vi "_s_Bronkhorst Serial Module.vi"(5 "Module (T:Enable)":bool=TRUE, 6 "Mode (T:Digital)":bool=TRUE, 7 "Command":T1=enum."Request Serial Number", 8 "error in (no error)":errorcluster, 9 "Setpoint %":dbl, 10 "Nodo":u8=3, 11 "VISA resource name":refnum<visa-resource-name>="COM1") -> (0 "error out":errorcluster, 1 "Reading":T2, 2 "Result":string, 3 "Value":string)   [LabVIEW 2013]
uses:
  _s_Bronkhorst Control.ctl
  <vilib>/Instr/_visa.llb/VISA Configure Serial Port (Instr).vi
panel:
  out "ReadString":string
  out "Bytes?":u32
  out "SendString":string
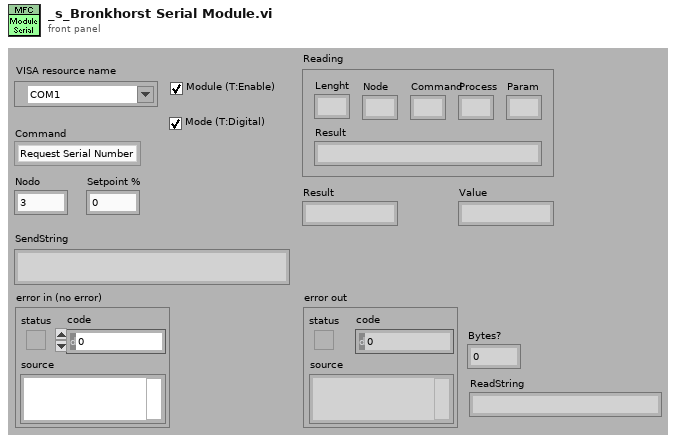
[diagram p1: front panel]
types:
  T1 = typedef "_s_Bronkhorst Control.ctl" = enum16{"Inicializar", "Request IdnString", "Request Serial Number", "Request Fluid Number", "Request Fluid Name", "Request Sensor Type", "Request Cap 0", "Request Cap100", "Request Units", "Request CapUnitStr", "Request Setpoint %", "Request Setpoint", "Request Measure %", "Request Measure ", "Send Control Mode", "Send Fluid Number", "Send Setpoint %", "Send Setpoint", "Shutdown"}
  T2 = cluster{"Lenght":string, "Node":string, "Process":string, "Param":string, "Command":string, "Result":string}
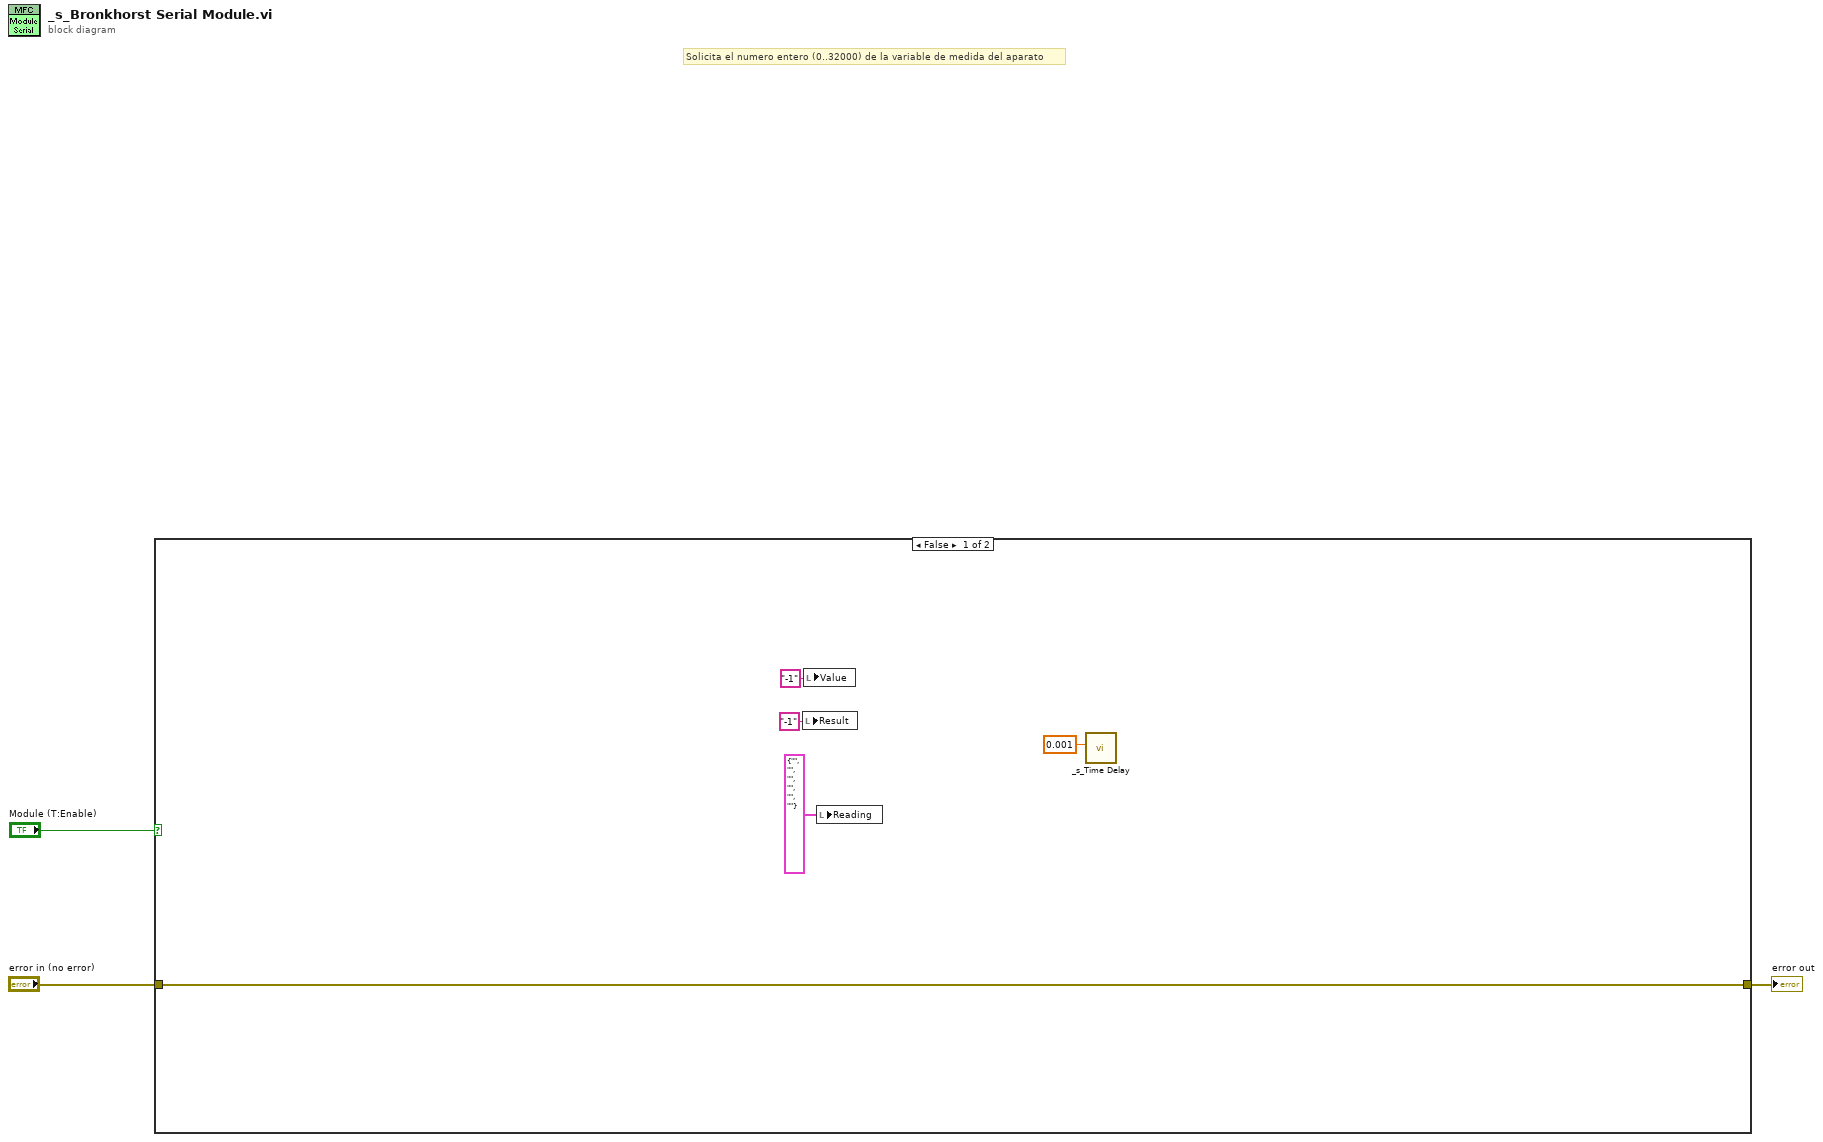
[diagram p0: block diagram]
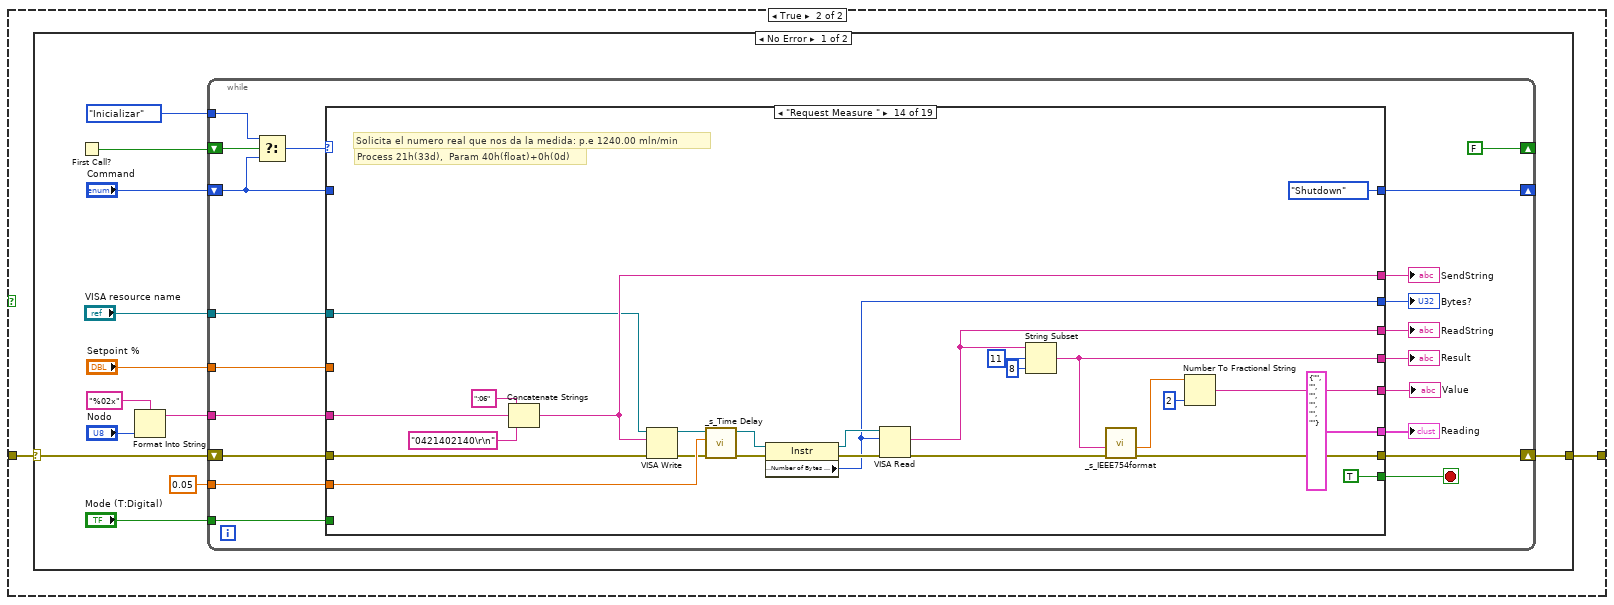
[diagram p2: hidden frame]
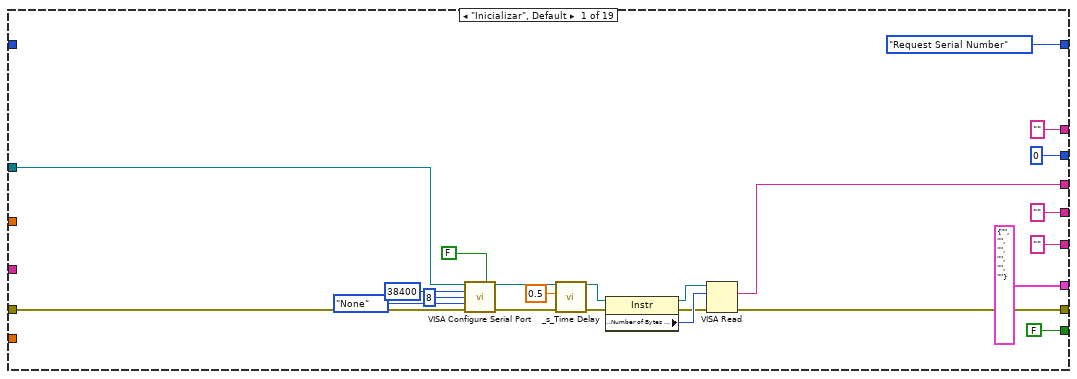
[diagram p3: hidden frame]
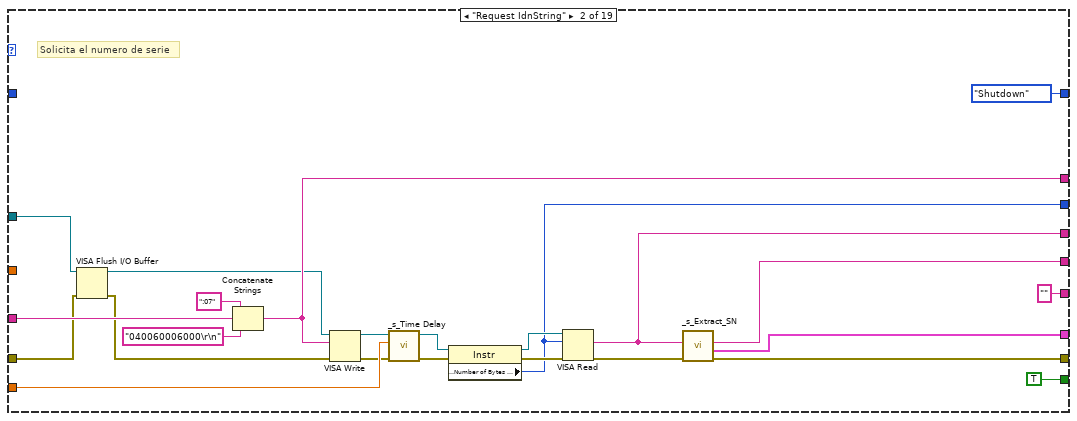
[diagram p4: hidden frame]
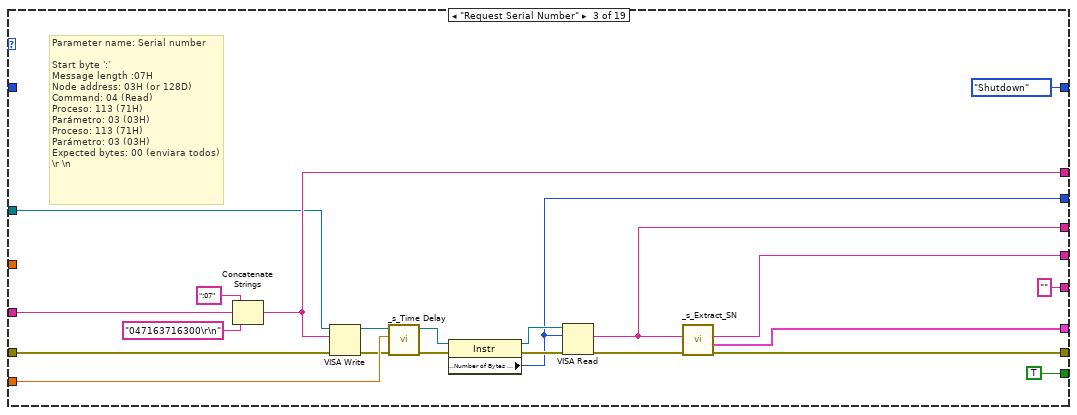
[diagram p5: hidden frame]
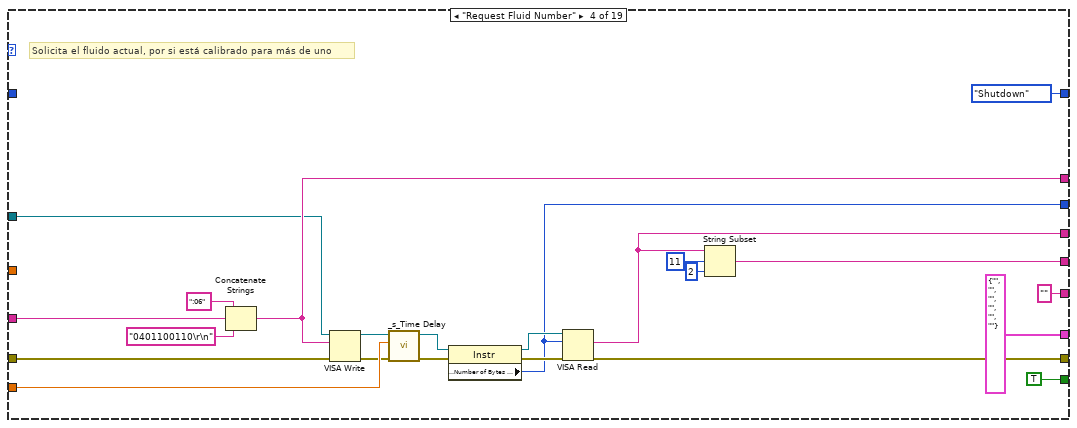
[diagram p6: hidden frame]
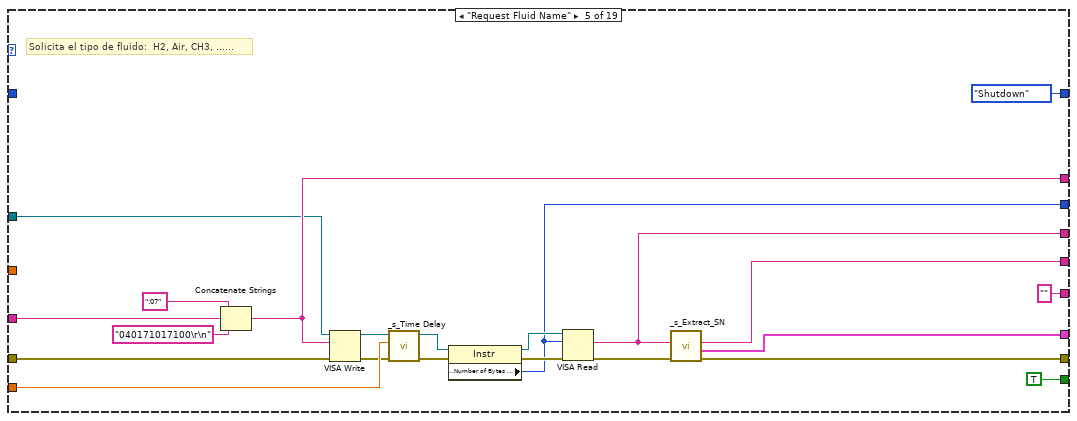
[diagram p7: hidden frame]
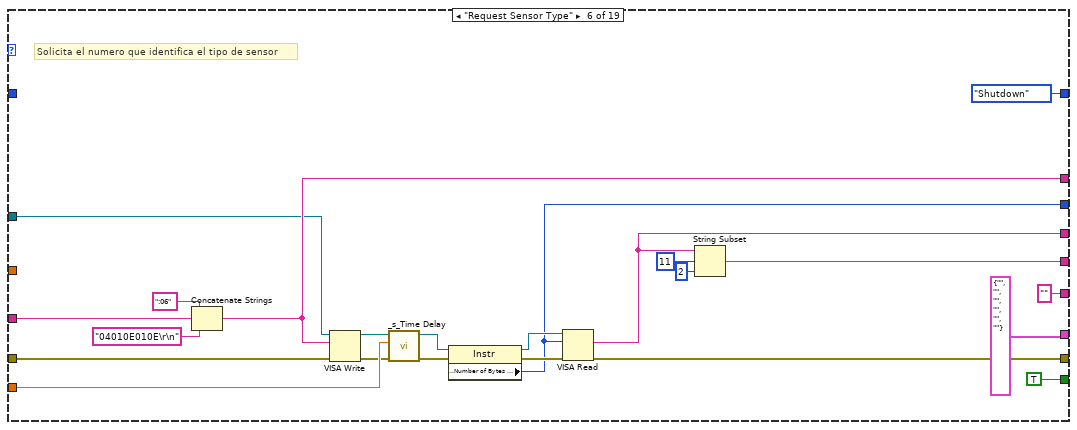
[diagram p8: hidden frame]
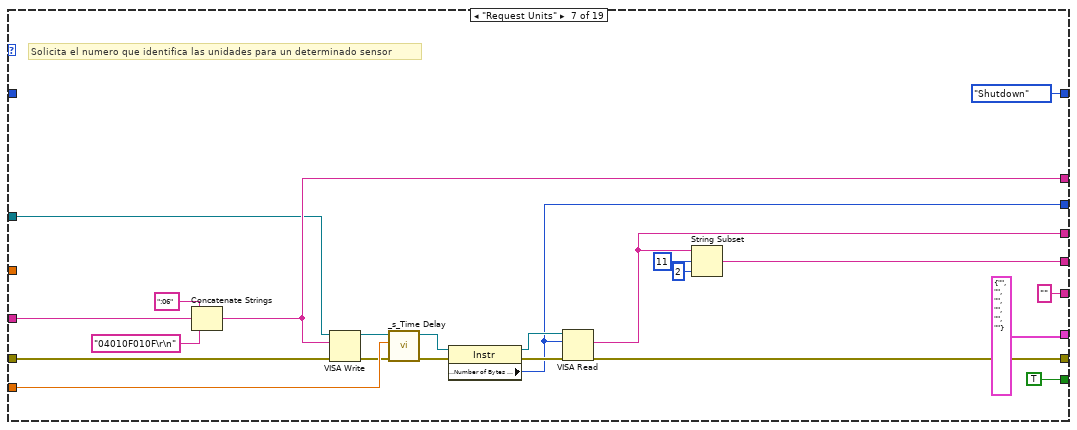
[diagram p9: hidden frame]
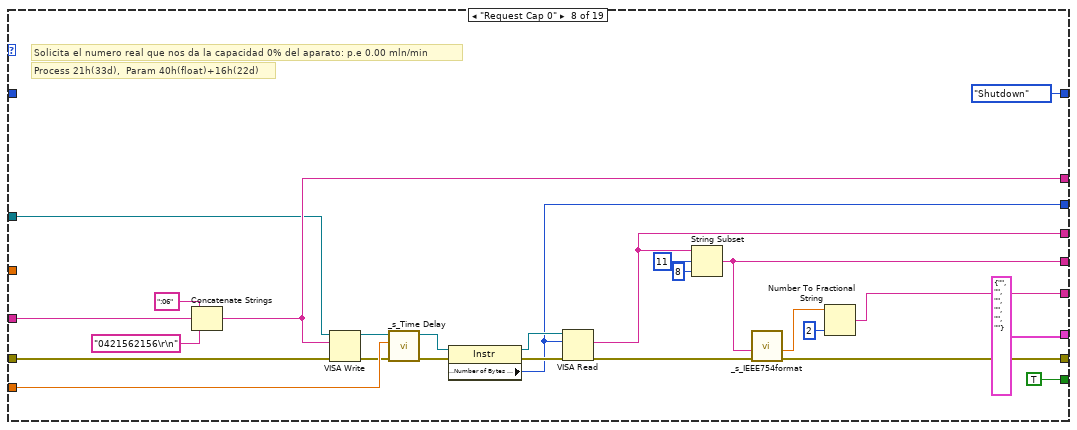
[diagram p10: hidden frame]
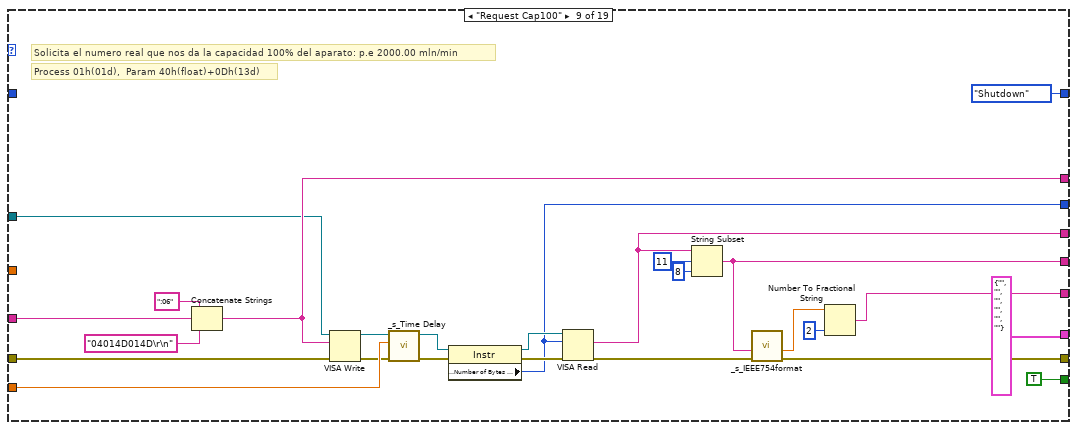
[diagram p11: hidden frame]
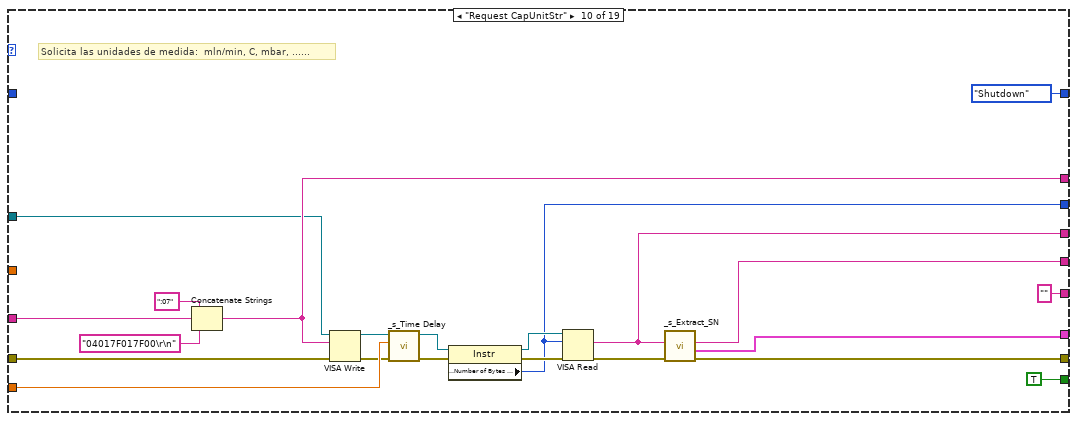
[diagram p12: hidden frame]
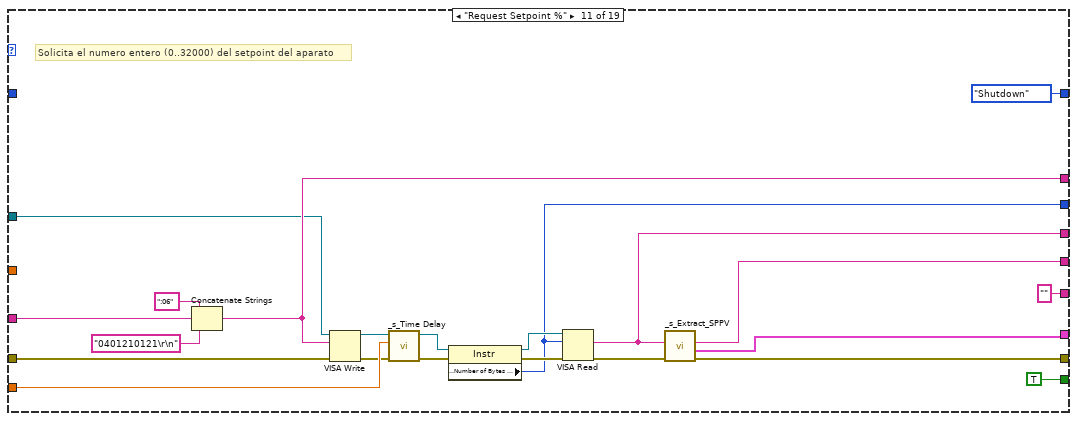
[diagram p13: hidden frame]
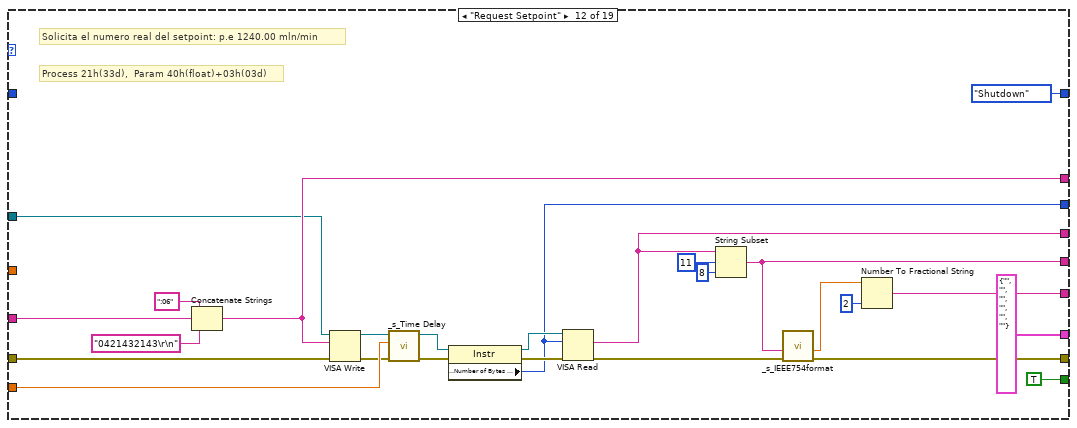
[diagram p14: hidden frame]
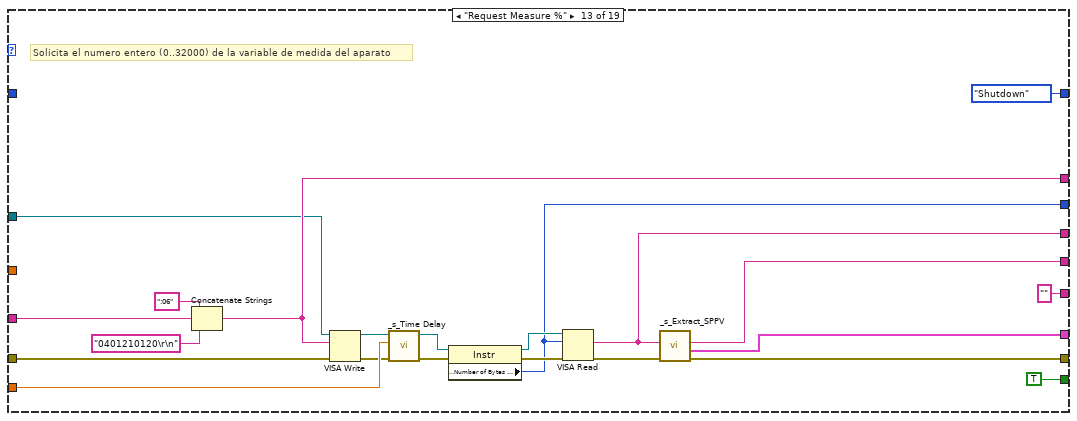
[diagram p15: hidden frame]
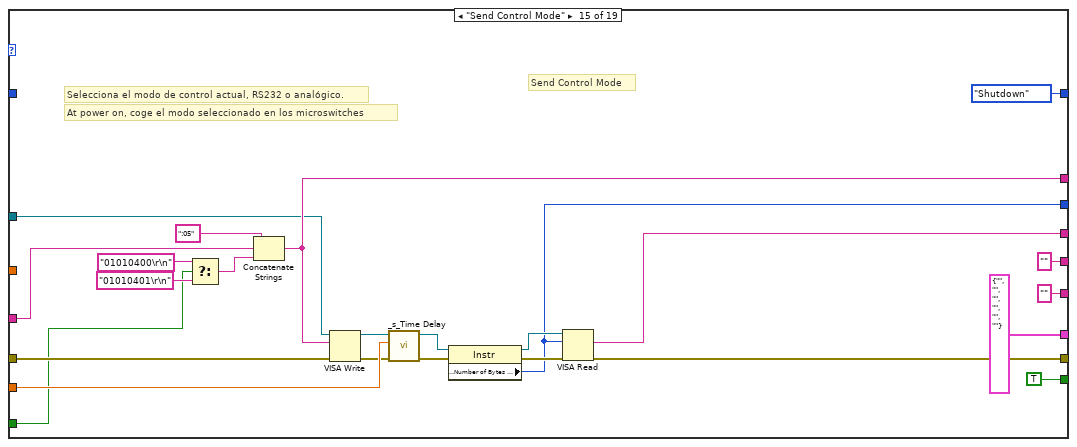
[diagram p16: hidden frame]
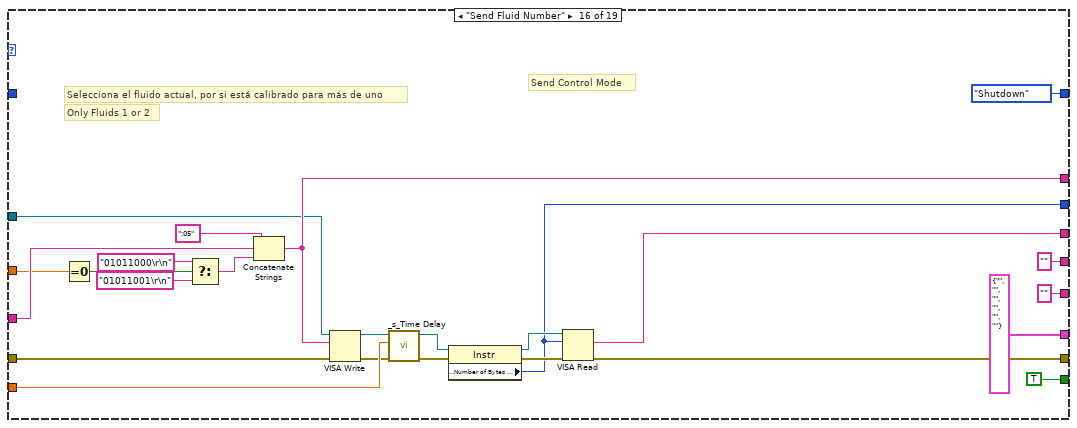
[diagram p17: hidden frame]
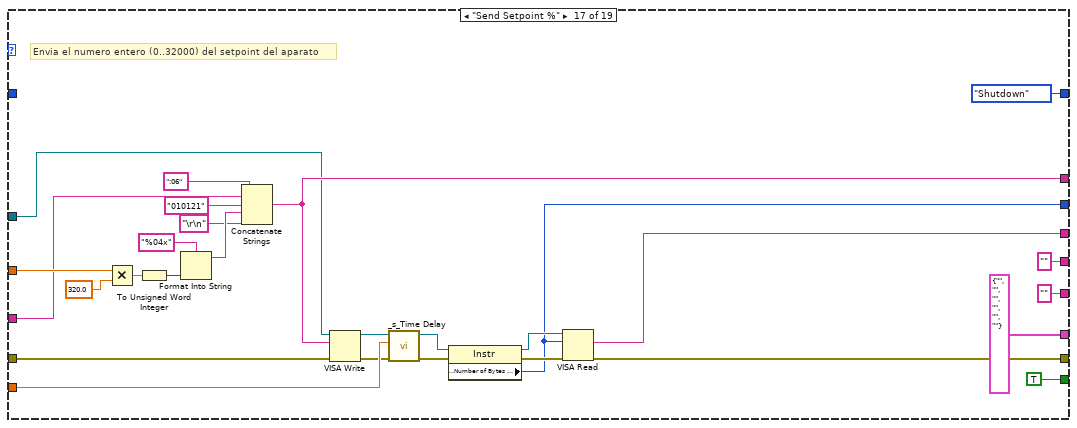
[diagram p18: hidden frame]
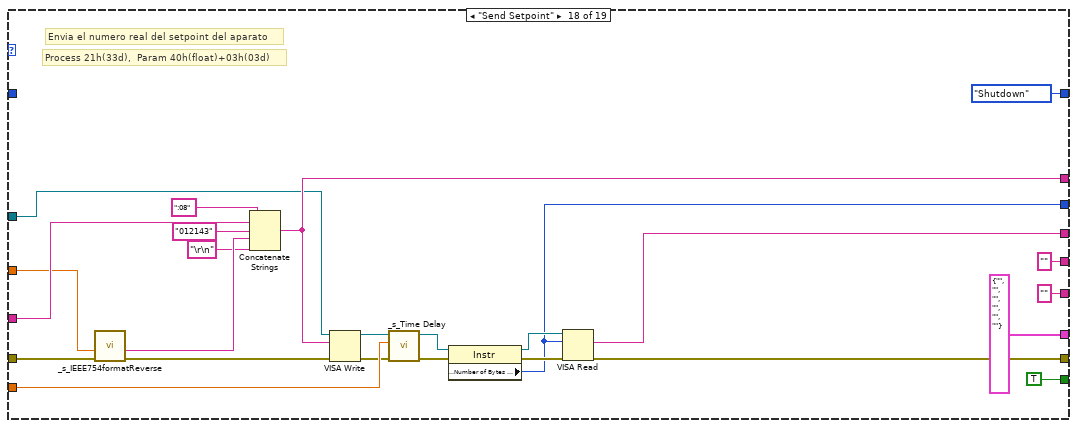
[diagram p19: hidden frame]
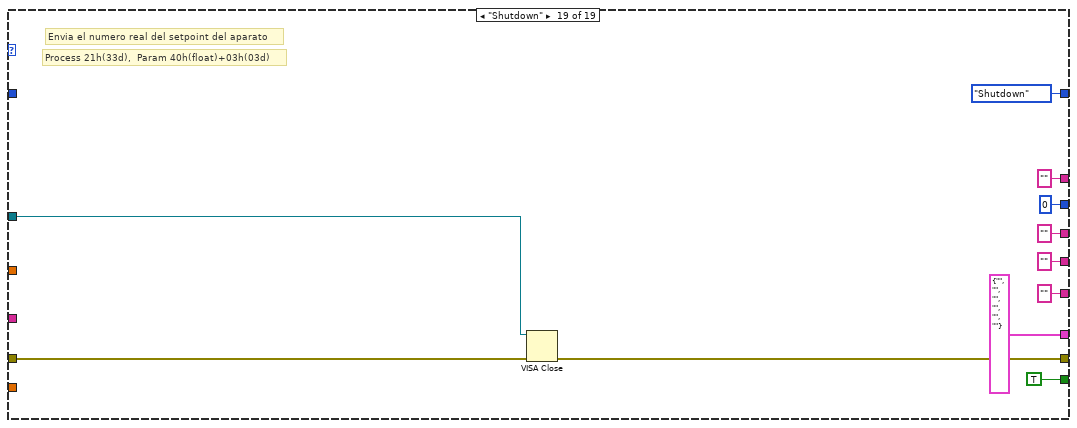
[diagram p20: hidden frame]
diagram:
  # "Solicita el numero entero (0..32000) de la variable de medida del aparato"
  n1 = case shown="False" "Module (T:Enable)" {
    tunnel: [w8 w10] -> w3
    tunnel: "error in (no error)" -> [w8 w9]
    frame False {
      n2 = local write "Result"("-1" ("read buffer")) -> ()
      n3 = local write "Value"("-1" ("read buffer")) -> ()
      n4 = local write "Reading"(T2 {"Lenght"="", "Node"="", "Process"="", "Param"="", "Command"="", "Result"=""} ("Reading")) -> ()
      n5 = call "_s_Time Delay.vi"("Delay Time (s)"=0.001) -> ()  [unwired: 10 in, 1 out]
    }
    frame True {
      n6 = case shown="No Error" w9 {
        selector: w9 -> [w21 w468]
        tunnel: [w20 w468] -> w10
        frame No Error {
          n7 = First Call?() -> (First Call?: T/F=w22:bool)
          n8 = Format Into String(format string="%02x", "Nodo") -> (resulting string=w15:string)  [unwired: 2 in, 1 out]
          n9 = while {
            shift-right: [w32] -> _
            shift-left: "Command" -> [w36]
            shift-right: [w38] -> w20
            shift-left: w21 -> [w39]
            shift-right: [FALSE ("First Call?: T/F")] -> _
            shift-left: w22 -> [w42]
            tunnel: _s_Bronkhorst_Control."Inicializar" ("Command") -> [w41]
            tunnel: 0.05 ("Delay Time (s)") -> [w31]
            tunnel: w15 -> [w30]
            tunnel: "Setpoint %" -> [w25]
            tunnel: "VISA resource name" -> [w24]
            tunnel: "Mode (T:Digital)" -> [w23]
            stop <- w40 stop-if-true
            n10 = Select(t=w41, s=w42, f=w36) -> (s? t:f=w33:T1)
            n11 = case shown="\"Request Measure \"" w33 {
              tunnel: [FALSE TRUE TRUE TRUE TRUE TRUE TRUE TRUE TRUE TRUE TRUE TRUE TRUE TRUE TRUE TRUE TRUE TRUE TRUE] -> w40
              tunnel: w39 -> [w58 w68 w102 w127 w148 w170 w192 w217 w242 w263 w284 w309 w330 w355 w378 w402 w429 w436 w461]
              tunnel: [w45 w83 w105 w113 w137 w155 w176 w199 w225 w249 w270 w291 w318 w337 w363 w385 w409 w445 w462] -> w38
              tunnel: w36 -> [_ _ _ _ _ _ _ _ _ _ _ _ _ _ _ _ _ _ _]
              tunnel: [w44 w74 w95 w114 w139 w157 w178 w202 w228 w251 w272 w295 w314 w340 w371 w395 w422 w447 "" ("read buffer")] -> w35
              tunnel: [u32 0 ("Bytes at Port") w71 w92 w121 w142 w164 w186 w211 w236 w257 w278 w303 w324 w349 w372 w396 w423 w448 u32 0 ("Bytes at Port")] -> w34
              tunnel: [_s_Bronkhorst_Control."Request Serial Number" ("Command") _s_Bronkhorst_Control."Shutdown" ("Command") _s_Bronkhorst_Control."Shutdown" ("Command") _s_Bronkhorst_Control."Shutdown" ("Command") _s_Bronkhorst_Control."Shutdown" ("Command") _s_Bronkhorst_Control."Shutdown" ("Command") _s_Bronkhorst_Control."Shutdown" ("Command") _s_Bronkhorst_Control."Shutdown" ("Command") _s_Bronkhorst_Control."Shutdown" ("Command") _s_Bronkhorst_Control."Shutdown" ("Command") _s_Bronkhorst_Control."Shutdown" ("Command") _s_Bronkhorst_Control."Shutdown" ("Command") _s_Bronkhorst_Control."Shutdown" ("Command") _s_Bronkhorst_Control."Shutdown" ("Command") _s_Bronkhorst_Control."Shutdown" ("Command") _s_Bronkhorst_Control."Shutdown" ("Command") _s_Bronkhorst_Control."Shutdown" ("Command") _s_Bronkhorst_Control."Shutdown" ("Command") _s_Bronkhorst_Control."Shutdown" ("Command")] -> w32
              tunnel: w31 -> [_ w85 w107 w130 w151 w173 w195 w220 w245 w266 w287 w312 w333 w358 w381 w405 w432 w456 _]
              tunnel: w30 -> [_ w84 w106 w117 w134 w161 w182 w207 w233 w254 w275 w300 w321 w346 w364 w387 w410 w438 _]
              tunnel: [T2 {"Lenght"="", "Node"="", "Process"="", "Param"="", "Command"="", "Result"=""} ("Reading") w73 w94 T2 {"Lenght"="", "Node"="", "Process"="", "Param"="", "Command"="", "Result"=""} ("Reading") w135 T2 {"Lenght"="", "Node"="", "Process"="", "Param"="", "Command"="", "Result"=""} ("Reading") T2 {"Lenght"="", "Node"="", "Process"="", "Param"="", "Command"="", "Result"=""} ("Reading") T2 {"Lenght"="", "Node"="", "Process"="", "Param"="", "Command"="", "Result"=""} ("Reading") T2 {"Lenght"="", "Node"="", "Process"="", "Param"="", "Command"="", "Result"=""} ("Reading") w247 w268 T2 {"Lenght"="", "Node"="", "Process"="", "Param"="", "Command"="", "Result"=""} ("Reading") w316 T2 {"Lenght"="", "Node"="", "Process"="", "Param"="", "Command"="", "Result"=""} ("Reading") T2 {"Lenght"="", "Node"="", "Process"="", "Param"="", "Command"="", "Result"=""} ("Reading") T2 {"Lenght"="", "Node"="", "Process"="", "Param"="", "Command"="", "Result"=""} ("Reading") T2 {"Lenght"="", "Node"="", "Process"="", "Param"="", "Command"="", "Result"=""} ("Reading") T2 {"Lenght"="", "Node"="", "Process"="", "Param"="", "Command"="", "Result"=""} ("Reading") T2 {"Lenght"="", "Node"="", "Process"="", "Param"="", "Command"="", "Result"=""} ("Reading")] -> w29
              tunnel: ["" ("Result") w72 w93 w112 w136 w156 w177 w197 w223 w248 w269 w289 w317 w336 "" ("read buffer") "" ("read buffer") "" ("read buffer") "" ("read buffer") "" ("read buffer")] -> w28
              tunnel: ["" w70 w91 w118 w133 w160 w181 w206 w232 w253 w274 w299 w320 w345 w365 w388 w412 w435 ""] -> w27
              tunnel: ["" "" "" "" "" "" "" w198 w224 "" "" w293 "" w339 "" "" "" "" ""] -> w26
              tunnel: w25 -> [_ _ _ _ _ _ _ _ _ _ _ _ _ _ _ w386 w411 w437 _]
              tunnel: w24 -> [w51 w65 w88 w109 w131 w152 w174 w196 w221 w246 w267 w288 w313 w334 w360 w382 w406 w433 w457]
              tunnel: w23 -> [_ _ _ _ _ _ _ _ _ _ _ _ _ _ w359 _ _ _ _]
              frame "Inicializar", Default {
                n12 = call-poly "VISA Configure Serial Port"("VISA resource name"=w51, "Enable Termination\nChar (T)"=FALSE ("Enable Termination\nChar (T)"), "baud rate (9600)"=u32 38400, "data bits (8)"=u16 8, "parity (0:none)"=enum16{"None", "Odd", "Even", "Mark", "Space"}."None", "error in (no error)"=w58) -> ("VISA resource name out"=w47:refnum<visa-resource-name>, "error out"=w57:errorcluster)  [unwired: 8 in]
                n13 = call "_s_Time Delay.vi"("error in (no error)"=w57, "Delay Time (s)"=0.5) -> ("error out"=w46:errorcluster)  [unwired: 9 in]
                n14 = property class="Instr"(reference=w47, error in=w46) -> (reference out=w48:refnum<visa-resource-name>, error out=w49:errorcluster, "Serial Settings:Number of Bytes at Serial Port"=w50:u32)
                n15 = VISA Read(VISA resource name=w48, byte count=w50, error in (no error)=w49) -> (read buffer=w44:string, error out=w45:errorcluster)  [unwired: 2 out]
              }
              frame "Request IdnString" {
                # "Solicita el numero de serie"
                n16 = VISA Flush I/O Buffer(VISA resource name=w65, error in (no error)=w68) -> (VISA resource name out=w66:refnum<visa-resource-name>, error out=w67:errorcluster)  [unwired: 1 in]
                n17 = Concatenate Strings(":07" ("string"), w84, "040060006000\r\n" ("string")) -> (w70:string)
                n18 = VISA Write(VISA resource name=w66, write buffer=w70, error in (no error)=w67) -> (VISA resource name out=w78:refnum<visa-resource-name>, error out=w80:errorcluster)  [unwired: 1 out]
                n19 = call "_s_Time Delay.vi"("error in (no error)"=w80, "Delay Time (s)"=w85) -> ("error out"=w79:errorcluster)  [unwired: 9 in]
                n20 = property class="Instr"(reference=w78, error in=w79) -> (reference out=w77:refnum<visa-resource-name>, error out=w75:errorcluster, "Serial Settings:Number of Bytes at Serial Port"=w71:u32)
                n21 = VISA Read(VISA resource name=w77, byte count=w71, error in (no error)=w75) -> (read buffer=w74:string, error out=w76:errorcluster)  [unwired: 2 out]
                n22 = call "_s_Extract_SN.vi"("error in (no error)"=w76, "Read String"=w74) -> ("error out"=w83:errorcluster, "Reading"=w73:T2, "Result"=w72:string)  [unwired: 7 in]
              }
              frame "Request Serial Number" {
                # "Parameter name: Serial number\n\nStart byte ':'\nMessage length :07H\nNode address: 03H (or 128D)\nCommand: 04 (Read)\nProceso: 113 (71H)\nParámetro: 03 (03H)\nProceso: 113 (71H)\nParámetro: 03 (03H)\nExpected bytes: 00 (enviara todos)\n\\r \\n"
                n23 = Concatenate Strings(":07" ("string"), w106, "047163716300\r\n" ("string")) -> (w91:string)
                n24 = VISA Write(VISA resource name=w88, write buffer=w91, error in (no error)=w102) -> (VISA resource name out=w99:refnum<visa-resource-name>, error out=w101:errorcluster)  [unwired: 1 out]
                n25 = call "_s_Time Delay.vi"("error in (no error)"=w101, "Delay Time (s)"=w107) -> ("error out"=w100:errorcluster)  [unwired: 9 in]
                n26 = property class="Instr"(reference=w99, error in=w100) -> (reference out=w98:refnum<visa-resource-name>, error out=w96:errorcluster, "Serial Settings:Number of Bytes at Serial Port"=w92:u32)
                n27 = VISA Read(VISA resource name=w98, byte count=w92, error in (no error)=w96) -> (read buffer=w95:string, error out=w97:errorcluster)  [unwired: 2 out]
                n28 = call "_s_Extract_SN.vi"("error in (no error)"=w97, "Read String"=w95) -> ("error out"=w105:errorcluster, "Reading"=w94:T2, "Result"=w93:string)  [unwired: 7 in]
              }
              frame "Request Fluid Number" {
                # "Solicita el fluido actual, por si está calibrado para más de uno"
                n29 = Concatenate Strings(":06" ("string"), w117, "0401100110\r\n" ("string")) -> (w118:string)
                n30 = VISA Write(VISA resource name=w109, write buffer=w118, error in (no error)=w127) -> (VISA resource name out=w124:refnum<visa-resource-name>, error out=w126:errorcluster)  [unwired: 1 out]
                n31 = call "_s_Time Delay.vi"("error in (no error)"=w126, "Delay Time (s)"=w130) -> ("error out"=w125:errorcluster)  [unwired: 9 in]
                n32 = property class="Instr"(reference=w124, error in=w125) -> (reference out=w123:refnum<visa-resource-name>, error out=w122:errorcluster, "Serial Settings:Number of Bytes at Serial Port"=w121:u32)
                n33 = VISA Read(VISA resource name=w123, byte count=w121, error in (no error)=w122) -> (read buffer=w114:string, error out=w113:errorcluster)  [unwired: 2 out]
                n34 = String Subset(string=w114, offset (0)=11, length (rest)=2 ("length (rest)")) -> (substring=w112:string)
              }
              frame "Request Fluid Name" {
                # "Solicita el tipo de fluido:  H2, Air, CH3, ......"
                n35 = Concatenate Strings(":07" ("string"), w134, "040171017100\r\n" ("string")) -> (w133:string)
                n36 = VISA Write(VISA resource name=w131, write buffer=w133, error in (no error)=w148) -> (VISA resource name out=w145:refnum<visa-resource-name>, error out=w147:errorcluster)  [unwired: 1 out]
                n37 = call "_s_Time Delay.vi"("error in (no error)"=w147, "Delay Time (s)"=w151) -> ("error out"=w146:errorcluster)  [unwired: 9 in]
                n38 = property class="Instr"(reference=w145, error in=w146) -> (reference out=w144:refnum<visa-resource-name>, error out=w143:errorcluster, "Serial Settings:Number of Bytes at Serial Port"=w142:u32)
                n39 = VISA Read(VISA resource name=w144, byte count=w142, error in (no error)=w143) -> (read buffer=w139:string, error out=w138:errorcluster)  [unwired: 2 out]
                n40 = call "_s_Extract_SN.vi"("error in (no error)"=w138, "Read String"=w139) -> ("error out"=w137:errorcluster, "Reading"=w135:T2, "Result"=w136:string)  [unwired: 7 in]
              }
              frame "Request Sensor Type" {
                # "Solicita el numero que identifica el tipo de sensor"
                n41 = Concatenate Strings(":06" ("string"), w161, "04010E010E\r\n" ("string")) -> (w160:string)
                n42 = VISA Write(VISA resource name=w152, write buffer=w160, error in (no error)=w170) -> (VISA resource name out=w167:refnum<visa-resource-name>, error out=w169:errorcluster)  [unwired: 1 out]
                n43 = call "_s_Time Delay.vi"("error in (no error)"=w169, "Delay Time (s)"=w173) -> ("error out"=w168:errorcluster)  [unwired: 9 in]
                n44 = property class="Instr"(reference=w167, error in=w168) -> (reference out=w166:refnum<visa-resource-name>, error out=w165:errorcluster, "Serial Settings:Number of Bytes at Serial Port"=w164:u32)
                n45 = VISA Read(VISA resource name=w166, byte count=w164, error in (no error)=w165) -> (read buffer=w157:string, error out=w155:errorcluster)  [unwired: 2 out]
                n46 = String Subset(string=w157, offset (0)=11, length (rest)=2 ("length (rest)")) -> (substring=w156:string)
              }
              frame "Request Units" {
                # "Solicita el numero que identifica las unidades para un determinado sensor"
                n47 = Concatenate Strings(":06" ("string"), w182, "04010F010F\r\n" ("string")) -> (w181:string)
                n48 = VISA Write(VISA resource name=w174, write buffer=w181, error in (no error)=w192) -> (VISA resource name out=w189:refnum<visa-resource-name>, error out=w191:errorcluster)  [unwired: 1 out]
                n49 = call "_s_Time Delay.vi"("error in (no error)"=w191, "Delay Time (s)"=w195) -> ("error out"=w190:errorcluster)  [unwired: 9 in]
                n50 = property class="Instr"(reference=w189, error in=w190) -> (reference out=w188:refnum<visa-resource-name>, error out=w187:errorcluster, "Serial Settings:Number of Bytes at Serial Port"=w186:u32)
                n51 = VISA Read(VISA resource name=w188, byte count=w186, error in (no error)=w187) -> (read buffer=w178:string, error out=w176:errorcluster)  [unwired: 2 out]
                n52 = String Subset(string=w178, offset (0)=11, length (rest)=2 ("length (rest)")) -> (substring=w177:string)
              }
              frame "Request Cap 0" {
                # "Process 21h(33d),  Param 40h(float)+16h(22d)"
                # "Solicita el numero real que nos da la capacidad 0% del aparato: p.e 0.00 mln/min"
                n53 = Concatenate Strings(":06" ("string"), w207, "0421562156\r\n" ("string")) -> (w206:string)
                n54 = VISA Write(VISA resource name=w196, write buffer=w206, error in (no error)=w217) -> (VISA resource name out=w214:refnum<visa-resource-name>, error out=w216:errorcluster)  [unwired: 1 out]
                n55 = call "_s_Time Delay.vi"("error in (no error)"=w216, "Delay Time (s)"=w220) -> ("error out"=w215:errorcluster)  [unwired: 9 in]
                n56 = property class="Instr"(reference=w214, error in=w215) -> (reference out=w213:refnum<visa-resource-name>, error out=w212:errorcluster, "Serial Settings:Number of Bytes at Serial Port"=w211:u32)
                n57 = VISA Read(VISA resource name=w213, byte count=w211, error in (no error)=w212) -> (read buffer=w202:string, error out=w201:errorcluster)  [unwired: 2 out]
                n58 = String Subset(string=w202, offset (0)=11, length (rest)=8 ("length (rest)")) -> (substring=w197:string)
                n59 = call "_s_IEEE754format.vi"("error in (no error)"=w201, "String"=w197) -> ("error out"=w199:errorcluster, "Number"=w200:sgl)  [unwired: 8 in]
                n60 = Number To Fractional String(number=w200, precision (6)=i16 2) -> (F-format string=w198:string)  [unwired: 2 in]
              }
              frame "Request Cap100" {
                # "Process 01h(01d),  Param 40h(float)+0Dh(13d)"
                # "Solicita el numero real que nos da la capacidad 100% del aparato: p.e 2000.00 mln/min"
                n61 = Concatenate Strings(":06" ("string"), w233, "04014D014D\r\n" ("string")) -> (w232:string)
                n62 = VISA Write(VISA resource name=w221, write buffer=w232, error in (no error)=w242) -> (VISA resource name out=w239:refnum<visa-resource-name>, error out=w241:errorcluster)  [unwired: 1 out]
                n63 = call "_s_Time Delay.vi"("error in (no error)"=w241, "Delay Time (s)"=w245) -> ("error out"=w240:errorcluster)  [unwired: 9 in]
                n64 = property class="Instr"(reference=w239, error in=w240) -> (reference out=w238:refnum<visa-resource-name>, error out=w237:errorcluster, "Serial Settings:Number of Bytes at Serial Port"=w236:u32)
                n65 = VISA Read(VISA resource name=w238, byte count=w236, error in (no error)=w237) -> (read buffer=w228:string, error out=w227:errorcluster)  [unwired: 2 out]
                n66 = String Subset(string=w228, offset (0)=11, length (rest)=8 ("length (rest)")) -> (substring=w223:string)
                n67 = call "_s_IEEE754format.vi"("error in (no error)"=w227, "String"=w223) -> ("error out"=w225:errorcluster, "Number"=w226:sgl)  [unwired: 8 in]
                n68 = Number To Fractional String(number=w226, precision (6)=i16 2) -> (F-format string=w224:string)  [unwired: 2 in]
              }
              frame "Request CapUnitStr" {
                # "Solicita las unidades de medida:  mln/min, C, mbar, ......"
                n69 = Concatenate Strings(":07" ("string"), w254, "04017F017F00\r\n" ("string")) -> (w253:string)
                n70 = VISA Write(VISA resource name=w246, write buffer=w253, error in (no error)=w263) -> (VISA resource name out=w260:refnum<visa-resource-name>, error out=w262:errorcluster)  [unwired: 1 out]
                n71 = call "_s_Time Delay.vi"("error in (no error)"=w262, "Delay Time (s)"=w266) -> ("error out"=w261:errorcluster)  [unwired: 9 in]
                n72 = property class="Instr"(reference=w260, error in=w261) -> (reference out=w259:refnum<visa-resource-name>, error out=w258:errorcluster, "Serial Settings:Number of Bytes at Serial Port"=w257:u32)
                n73 = VISA Read(VISA resource name=w259, byte count=w257, error in (no error)=w258) -> (read buffer=w251:string, error out=w250:errorcluster)  [unwired: 2 out]
                n74 = call "_s_Extract_SN.vi"("error in (no error)"=w250, "Read String"=w251) -> ("error out"=w249:errorcluster, "Reading"=w247:T2, "Result"=w248:string)  [unwired: 7 in]
              }
              frame "Request Setpoint %" {
                # "Solicita el numero entero (0..32000) del setpoint del aparato"
                n75 = Concatenate Strings(":06" ("string"), w275, "0401210121\r\n" ("string")) -> (w274:string)
                n76 = VISA Write(VISA resource name=w267, write buffer=w274, error in (no error)=w284) -> (VISA resource name out=w281:refnum<visa-resource-name>, error out=w283:errorcluster)  [unwired: 1 out]
                n77 = call "_s_Time Delay.vi"("error in (no error)"=w283, "Delay Time (s)"=w287) -> ("error out"=w282:errorcluster)  [unwired: 9 in]
                n78 = property class="Instr"(reference=w281, error in=w282) -> (reference out=w280:refnum<visa-resource-name>, error out=w279:errorcluster, "Serial Settings:Number of Bytes at Serial Port"=w278:u32)
                n79 = VISA Read(VISA resource name=w280, byte count=w278, error in (no error)=w279) -> (read buffer=w272:string, error out=w271:errorcluster)  [unwired: 2 out]
                n80 = call "_s_Extract_SPPV.vi"("error in (no error)"=w271, "Read String"=w272) -> ("error out"=w270:errorcluster, "Reading"=w268:T2, "Setpoint"=w269:string)  [unwired: 7 in]
              }
              frame "Request Setpoint" {
                # "Process 21h(33d),  Param 40h(float)+03h(03d)"
                # "Solicita el numero real del setpoint: p.e 1240.00 mln/min"
                n81 = Concatenate Strings(":06" ("string"), w300, "0421432143\r\n" ("string")) -> (w299:string)
                n82 = VISA Write(VISA resource name=w288, write buffer=w299, error in (no error)=w309) -> (VISA resource name out=w306:refnum<visa-resource-name>, error out=w308:errorcluster)  [unwired: 1 out]
                n83 = call "_s_Time Delay.vi"("error in (no error)"=w308, "Delay Time (s)"=w312) -> ("error out"=w307:errorcluster)  [unwired: 9 in]
                n84 = property class="Instr"(reference=w306, error in=w307) -> (reference out=w305:refnum<visa-resource-name>, error out=w304:errorcluster, "Serial Settings:Number of Bytes at Serial Port"=w303:u32)
                n85 = VISA Read(VISA resource name=w305, byte count=w303, error in (no error)=w304) -> (read buffer=w295:string, error out=w296:errorcluster)  [unwired: 2 out]
                n86 = String Subset(string=w295, offset (0)=11, length (rest)=8 ("length (rest)")) -> (substring=w289:string)
                n87 = call "_s_IEEE754format.vi"("error in (no error)"=w296, "String"=w289) -> ("error out"=w291:errorcluster, "Number"=w290:sgl)  [unwired: 8 in]
                n88 = Number To Fractional String(number=w290, precision (6)=i16 2) -> (F-format string=w293:string)  [unwired: 2 in]
              }
              frame "Request Measure %" {
                # "Solicita el numero entero (0..32000) de la variable de medida del aparato"
                n89 = Concatenate Strings(":06" ("string"), w321, "0401210120\r\n" ("string")) -> (w320:string)
                n90 = VISA Write(VISA resource name=w313, write buffer=w320, error in (no error)=w330) -> (VISA resource name out=w327:refnum<visa-resource-name>, error out=w329:errorcluster)  [unwired: 1 out]
                n91 = call "_s_Time Delay.vi"("error in (no error)"=w329, "Delay Time (s)"=w333) -> ("error out"=w328:errorcluster)  [unwired: 9 in]
                n92 = property class="Instr"(reference=w327, error in=w328) -> (reference out=w326:refnum<visa-resource-name>, error out=w325:errorcluster, "Serial Settings:Number of Bytes at Serial Port"=w324:u32)
                n93 = VISA Read(VISA resource name=w326, byte count=w324, error in (no error)=w325) -> (read buffer=w314:string, error out=w319:errorcluster)  [unwired: 2 out]
                n94 = call "_s_Extract_SPPV.vi"("error in (no error)"=w319, "Read String"=w314) -> ("error out"=w318:errorcluster, "Reading"=w316:T2, "Setpoint"=w317:string)  [unwired: 7 in]
              }
              frame "Request Measure " {
                # "Process 21h(33d),  Param 40h(float)+0h(0d)"
                # "Solicita el numero real que nos da la medida: p.e 1240.00 mln/min"
                n95 = Concatenate Strings(":06" ("string"), w346, "0421402140\r\n" ("string")) -> (w345:string)
                n96 = VISA Write(VISA resource name=w334, write buffer=w345, error in (no error)=w355) -> (VISA resource name out=w352:refnum<visa-resource-name>, error out=w354:errorcluster)  [unwired: 1 out]
                n97 = call "_s_Time Delay.vi"("error in (no error)"=w354, "Delay Time (s)"=w358) -> ("error out"=w353:errorcluster)  [unwired: 9 in]
                n98 = property class="Instr"(reference=w352, error in=w353) -> (reference out=w351:refnum<visa-resource-name>, error out=w350:errorcluster, "Serial Settings:Number of Bytes at Serial Port"=w349:u32)
                n99 = VISA Read(VISA resource name=w351, byte count=w349, error in (no error)=w350) -> (read buffer=w340:string, error out=w338:errorcluster)  [unwired: 2 out]
                n100 = String Subset(string=w340, offset (0)=11, length (rest)=8 ("length (rest)")) -> (substring=w336:string)
                n101 = call "_s_IEEE754format.vi"("error in (no error)"=w338, "String"=w336) -> ("error out"=w337:errorcluster, "Number"=w344:sgl)  [unwired: 8 in]
                n102 = Number To Fractional String(number=w344, precision (6)=i16 2) -> (F-format string=w339:string)  [unwired: 2 in]
              }
              frame "Send Control Mode" {
                # "Send Control Mode"
                # "Selecciona el modo de control actual, RS232 o analógico."
                # "At power on, coge el modo seleccionado en los microswitches"
                n103 = Select(t="01010400\r\n" ("string"), s=w359, f="01010401\r\n" ("string")) -> (s? t:f=w367:string)
                n104 = Concatenate Strings(":05" ("string"), w364, w367) -> (w365:string)
                n105 = VISA Write(VISA resource name=w360, write buffer=w365, error in (no error)=w378) -> (VISA resource name out=w375:refnum<visa-resource-name>, error out=w377:errorcluster)  [unwired: 1 out]
                n106 = call "_s_Time Delay.vi"("error in (no error)"=w377, "Delay Time (s)"=w381) -> ("error out"=w376:errorcluster)  [unwired: 9 in]
                n107 = property class="Instr"(reference=w375, error in=w376) -> (reference out=w374:refnum<visa-resource-name>, error out=w373:errorcluster, "Serial Settings:Number of Bytes at Serial Port"=w372:u32)
                n108 = VISA Read(VISA resource name=w374, byte count=w372, error in (no error)=w373) -> (read buffer=w371:string, error out=w363:errorcluster)  [unwired: 2 out]
              }
              frame "Send Fluid Number" {
                # "Send Control Mode"
                # "Selecciona el fluido actual, por si está calibrado para más de uno"
                # "Only Fluids 1 or 2"
                n109 = Equal To 0?(x=w386) -> (x = 0?=w390:bool)
                n110 = Select(t="01011000\r\n" ("string"), s=w390, f="01011001\r\n" ("string")) -> (s? t:f=w391:string)
                n111 = Concatenate Strings(":05" ("string"), w387, w391) -> (w388:string)
                n112 = VISA Write(VISA resource name=w382, write buffer=w388, error in (no error)=w402) -> (VISA resource name out=w399:refnum<visa-resource-name>, error out=w401:errorcluster)  [unwired: 1 out]
                n113 = call "_s_Time Delay.vi"("error in (no error)"=w401, "Delay Time (s)"=w405) -> ("error out"=w400:errorcluster)  [unwired: 9 in]
                n114 = property class="Instr"(reference=w399, error in=w400) -> (reference out=w398:refnum<visa-resource-name>, error out=w397:errorcluster, "Serial Settings:Number of Bytes at Serial Port"=w396:u32)
                n115 = VISA Read(VISA resource name=w398, byte count=w396, error in (no error)=w397) -> (read buffer=w395:string, error out=w385:errorcluster)  [unwired: 2 out]
              }
              frame "Send Setpoint %" {
                # "Envia el numero entero (0..32000) del setpoint del aparato"
                n116 = Multiply(x=w411, y=320.0) -> (x*y=w417:dbl)
                n117 = To Unsigned Word Integer(number=w417) -> (unsigned 16bit integer=w418:u16)
                n118 = Format Into String(format string="%04x", w418) -> (resulting string=w420:string)  [unwired: 2 in, 1 out]
                n119 = Concatenate Strings(":06" ("string"), w410, "010121" ("string"), w420, "\r\n" ("string")) -> (w412:string)
                n120 = VISA Write(VISA resource name=w406, write buffer=w412, error in (no error)=w429) -> (VISA resource name out=w426:refnum<visa-resource-name>, error out=w428:errorcluster)  [unwired: 1 out]
                n121 = call "_s_Time Delay.vi"("error in (no error)"=w428, "Delay Time (s)"=w432) -> ("error out"=w427:errorcluster)  [unwired: 9 in]
                n122 = property class="Instr"(reference=w426, error in=w427) -> (reference out=w425:refnum<visa-resource-name>, error out=w424:errorcluster, "Serial Settings:Number of Bytes at Serial Port"=w423:u32)
                n123 = VISA Read(VISA resource name=w425, byte count=w423, error in (no error)=w424) -> (read buffer=w422:string, error out=w409:errorcluster)  [unwired: 2 out]
              }
              frame "Send Setpoint" {
                # "Process 21h(33d),  Param 40h(float)+03h(03d)"
                # "Envia el numero real del setpoint del aparato"
                n124 = call "_s_IEEE754formatReverse.vi"("error in (no error)"=w436, "Number"=w437) -> ("error out"=w434:errorcluster, "String"=w442:string)  [unwired: 8 in]
                n125 = Concatenate Strings(":08" ("string"), w438, "012143" ("string"), w442, "\r\n" ("string")) -> (w435:string)
                n126 = VISA Write(VISA resource name=w433, write buffer=w435, error in (no error)=w434) -> (VISA resource name out=w451:refnum<visa-resource-name>, error out=w453:errorcluster)  [unwired: 1 out]
                n127 = call "_s_Time Delay.vi"("error in (no error)"=w453, "Delay Time (s)"=w456) -> ("error out"=w452:errorcluster)  [unwired: 9 in]
                n128 = property class="Instr"(reference=w451, error in=w452) -> (reference out=w450:refnum<visa-resource-name>, error out=w449:errorcluster, "Serial Settings:Number of Bytes at Serial Port"=w448:u32)
                n129 = VISA Read(VISA resource name=w450, byte count=w448, error in (no error)=w449) -> (read buffer=w447:string, error out=w445:errorcluster)  [unwired: 2 out]
              }
              frame "Shutdown" {
                # "Process 21h(33d),  Param 40h(float)+03h(03d)"
                # "Envia el numero real del setpoint del aparato"
                n130 = VISA Close(VISA resource name=w457, error in (no error)=w461) -> (error out=w462:errorcluster)
              }
            }
            "ReadString" <- w35
            "Bytes?" <- w34
            "Result" <- w28
            "Reading" <- w29
            "SendString" <- w27
            "Value" <- w26
          }
        }
        frame Error {
        }
      }
    }
  }
  "error out" <- w3
